vi "My Nonlinear Curve Fit TRDL bounds.vi"(0 "Y":dbl[](array[numeric]), 1 "f(x,a)":T4, 2 "data":variant, 5 "X":dbl[](array[numeric]), 7 "Weight":dbl[](array[numeric]), 9 "initial parameters":dbl[](array[numeric]), 11 "error in (no error)":errorcluster, 12 "termination":cluster{"max iteration":i32, "tolerance":dbl}={"max iteration"=200, "tolerance"=1e-08}, 13 "parameter bounds":T3, 14 "method":T2 items=["Least Square", "Least Absolute Residual", "Bisquare"]) -> (3 "Fit Aborted?":bool, 4 "best nonlinear fit":dbl[](array[numeric]), 6 "best fit parameters":dbl[](array[numeric]), 8 "covariance":T5, 10 "Fit Statistics":T1, 15 "error out":errorcluster)   [LabVIEW 2019]
uses:
  <vilib>/Analysis/Matrix/Datatypes/RealMatrix.ctl
  <vilib>/gmath/NumericalOptimization/LM model function reference.ctl
  <vilib>/Analysis/6fits.llb/Curve Fitting Criteria.ctl
  Fit Statistics.ctl
  <vilib>/gmath/NumericalOptimization/LM model function.ctl
  My Fit Stopping Criteria.ctl
  <vilib>/gmath/NumericalOptimization/LM_output select.ctl
  Abort Fit Global.vi
  <vilib>/gmath/NI_Gmath.lvlib
  <vilib>/Analysis/NI_AALBase.lvlib
  <vilib>/Analysis/Matrix/NI_Matrix.lvlib
  <vilib>/Analysis/NI_AALPro.lvlib
panel:
  out "Waveform Graph":dbl[](graph)
  in  "Delay (ms)":i32
  in  "Debug":bool
  out "Parameters Chart":dbl[][](graph)
  out "Function & Fit Graph":cluster{"New Coefficients":dbl[]}[](graph)
  in  "TR update constants":cluster{"h1":dbl, "h2":dbl, "a1":dbl, "a2":dbl}={"h1"=0.0001, "h2"=0.99, "a1"=0.25, "a2"=3.5}
  out "number of function calls":i32
  out "residue":dbl
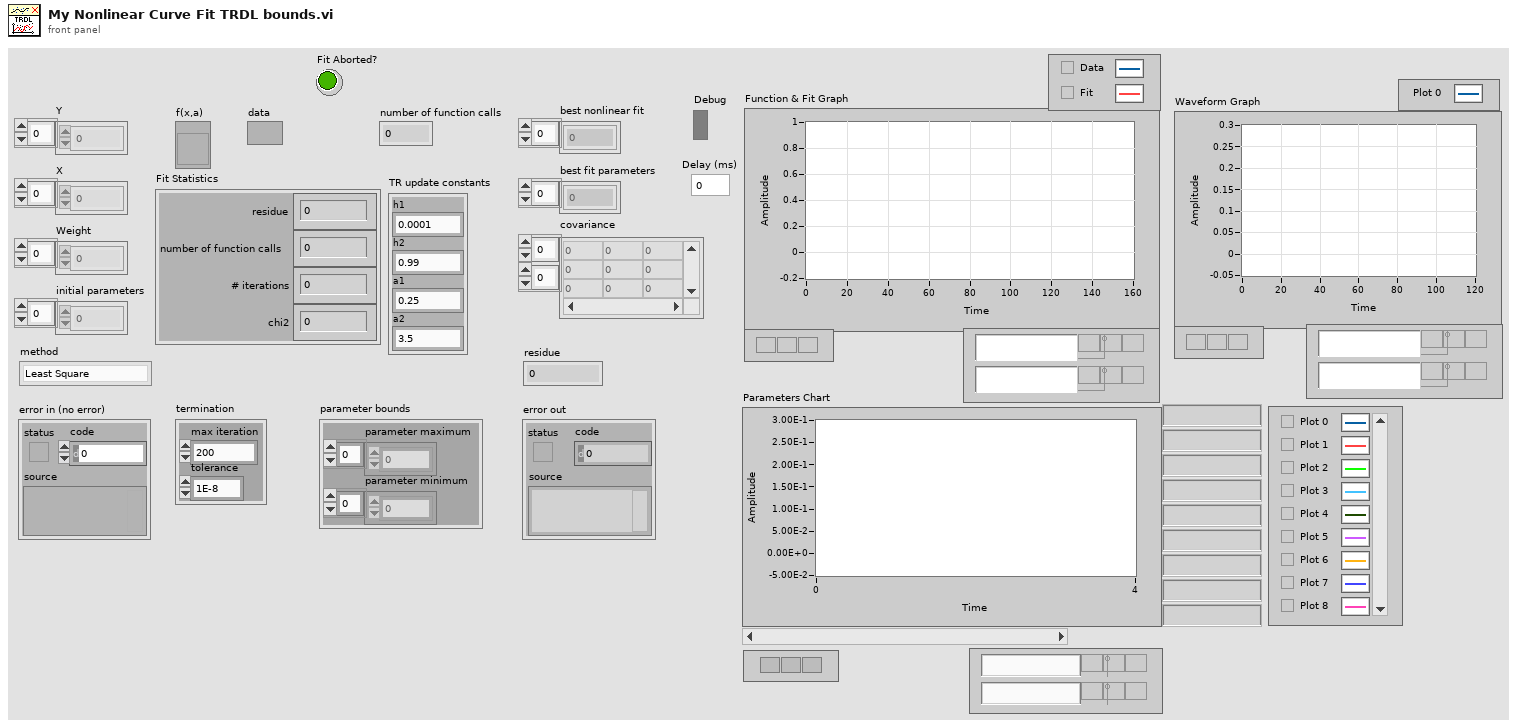
[diagram p1: front panel]
types:
  T1 = typedef "Fit Statistics.ctl" = cluster{"# iterations":i32, "number of function calls":i32, "chi2":dbl, "residue":dbl}
  T2 = typedef "NI_AALPro.lvlib/Curve Fitting Criteria.ctl" = u16
  T3 = cluster{"parameter minimum":dbl[], "parameter maximum":dbl[]}
  T4 = typedef "NI_Gmath.lvlib/LM model function reference.ctl" = refnum<vi>
  T5 = typedef "NI_Matrix.lvlib/RealMatrix.ctl" = dbl[][]
  T6 = typedef "My Fit Stopping Criteria.ctl" = cluster{"function tolerance":dbl, "parameter tolerance":dbl, "max iterations":i32, "max function calls":i32, "gradient tolerance":dbl, "max time (sec)":dbl, "initial tick count":u32, "min lambda":dbl, "max lambda":dbl}
  T7 = typedef "NI_Gmath.lvlib/LM model function.ctl" = cluster{"f(x,a)":T4, "data":variant}
  T8 = typedef "NI_Gmath.lvlib/LM_output select.ctl" = cluster{"model function":bool, "gradient":bool}
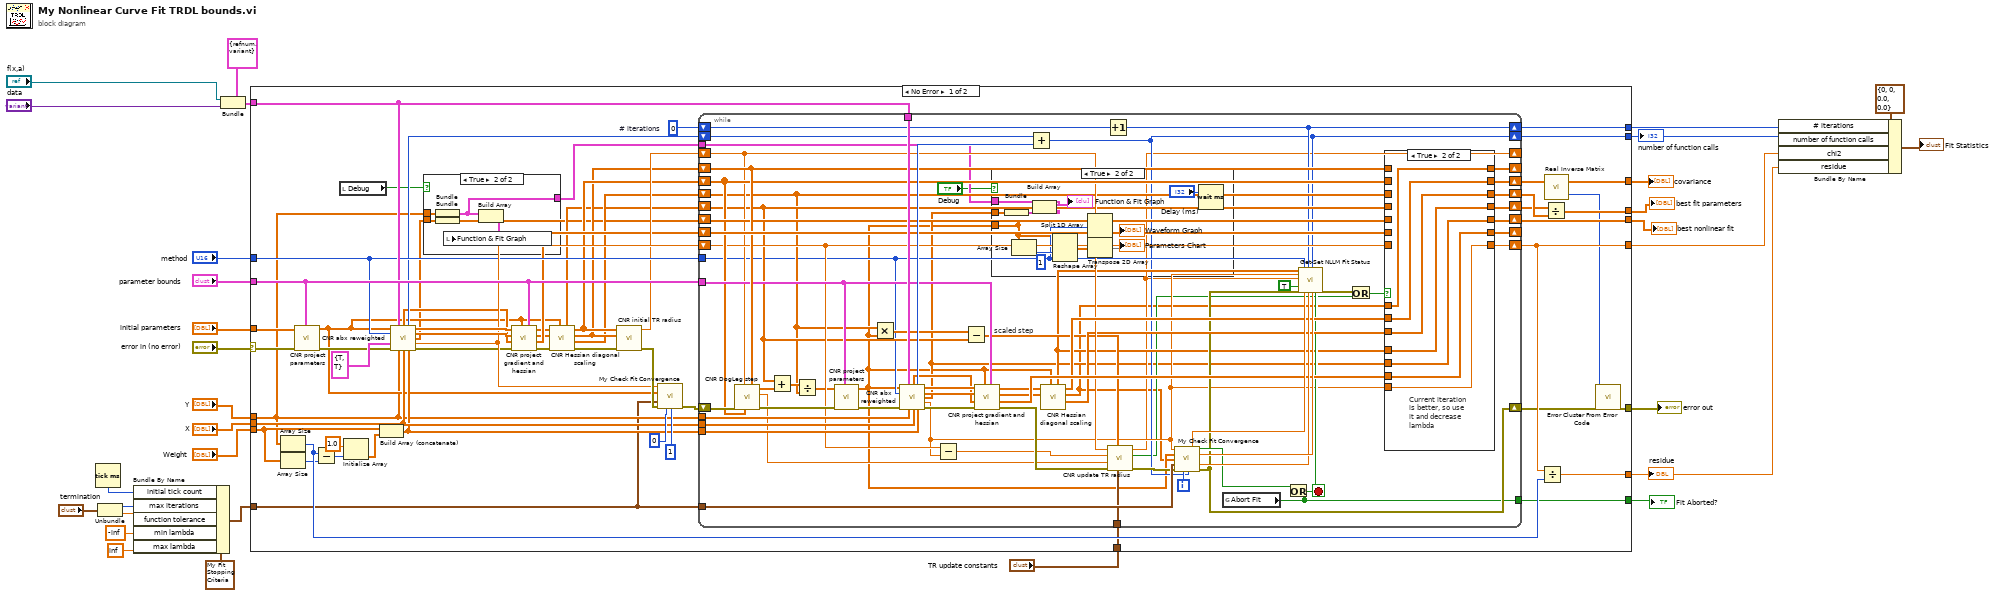
[diagram p0: block diagram]
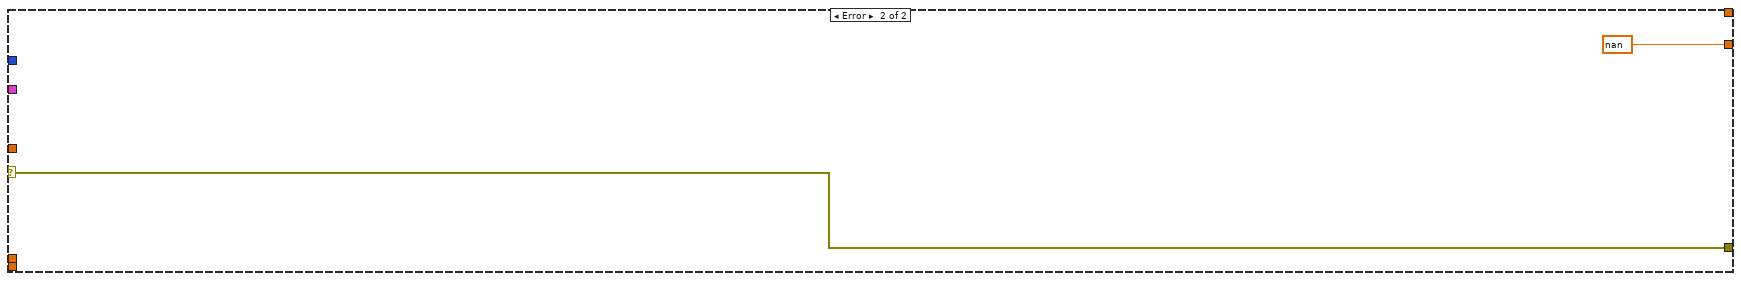
[diagram p5: hidden frame]
diagram:
  n1 = Tick Count (ms)() -> (millisecond timer value=w3:u32)
  n2 = Unbundle("termination") -> ("max iteration"=w21:i32, "tolerance"=w12:dbl)
  n3 = Bundle By Name(cluster=T6 {"function tolerance"=1e-06, "parameter tolerance"=100000000.0, "max iterations"=0, "max function calls"=1000000000, "gradient tolerance"=100000000.0, "max time (sec)"=-1.0, "initial tick count"=0, "min lambda"=1e-06, "max lambda"=1e-06} ("my stopping criteria"), "initial tick count"=w3, "max iterations"=w21, "function tolerance"=w12, "min lambda"=-inf, "max lambda"=inf) -> (w17:T6)
  n4 = Bundle(cluster=T7 {"f(x,a)"=refnum, "data"=variant} ("model function"), "f(x,a)"="f(x,a)", "data"="data") -> (w18:T7)
  n5 = case shown="No Error" "error in (no error)" {
    selector: "error in (no error)" -> [w72 w188]
    tunnel: [w44 _] -> w31
    tunnel: [w86 _] -> w7
    tunnel: "initial parameters" -> [w48 _]
    tunnel: [w58 _] -> w29
    tunnel: [w73 _] -> w28
    tunnel: "Weight" -> [w81 _]
    tunnel: "Y" -> [w34 _]
    tunnel: w17 -> [w32 _]
    tunnel: "X" -> [w60 _]
    tunnel: [w39 w188] -> w24
    tunnel: w18 -> [w66 _]
    tunnel: [w77 _] -> w8
    tunnel: "parameter bounds" -> [w71 _]
    tunnel: "method" -> [w65 _]
    tunnel: "TR update constants" -> [w57 _]
    tunnel: [w42 _] -> w10
    tunnel: [w41 nan ("chiSqr")] -> w6
    tunnel: [w37 _] -> w4
    frame No Error {
      w43 = 0  # # iterations
      n6 = Array Size(array=w34) -> (size(s)=w87:i32)
      n7 = Array Size(array=w81) -> (size(s)=w84:i32)
      n8 = call <vilib>:"CNR project parameters.vi"("bounds"=w71, "error in"=w72, "parameters"=w48) -> ("error out"=w64:errorcluster, "projected parameters"=w47:dbl[])  [unwired: 7 out]
      n9 = Subtract(x=w87, y=w84) -> (x-y=w83:i32)
      n10 = local read "Debug"() -> (w36:bool)
      n11 = Initialize Array(1.0, w83) -> (w82:dbl[])
      n12 = Build Array (concatenate)(w81, w82) -> (w59:dbl[])
      n13 = call <vilib>:"CNR abx reweighted.vi"("parameters"=w47, "model function"=w66, "method"=w65, "output control"=T8 {"model function"=TRUE, "gradient"=TRUE}, "error in (no error)"=w64, "Y"=w34, "X"=w60, "Weight"=w59) -> ("Jacobian"=w55:T5, "number of function calls"=w63:i32, "Hessian"=w70:T5, "gradient"=w69:dbl[], "best fit"=w35:dbl[], "chiSqr"=w68:dbl, "error out"=w62:errorcluster)  [unwired: 1 in]
      n14 = case shown="True" w36 {
        tunnel: w35 -> [_ w91]
        tunnel: w34 -> [_ w90]
        tunnel: [_ w88] -> w33
        frame False {
        }
        frame True {
          n15 = Bundle("Y"=w90) -> (w88:cluster{"Y":dbl[]})  [unwired: 1 in]
          n16 = Bundle("best fit"=w91) -> (w92:cluster{"best fit":dbl[]})  [unwired: 1 in]
          n17 = Build Array(w88, w92) -> (w89:cluster{"best fit":dbl[]}[])
          n18 = local write "Function & Fit Graph"(w89) -> ()
        }
      }
      n19 = call <vilib>:"CNR project gradient and hessian.vi"("bounds"=w71, "projected parameters"=w47, "error in"=w62, "Jacobian"=w55, "gradient"=w69, "Hessian"=w70) -> ("error out"=w61:errorcluster, "projected jacobian"=w54:T5, "projected gradient"=w51:dbl[], "projected Hessian"=w53:T5)  [unwired: 1 in, 1 out]
      n20 = call <vilib>:"CNR Hessian diagonal scaling.vi"("parameters"=w47, "gradient"=w51, "Hessian"=w53) -> ("D"=w49:dbl[], "scaled gradient"=w50:dbl[], "scaled Hessian"=w52:T5, "scaled parameters"=w46:dbl[])  [unwired: 5 out]
      n21 = call <vilib>:"CNR initial TR radius.vi"("error in"=w61, "g"=w50, "H"=w52) -> ("error out"=w75:errorcluster, "initial TR radius"=w56:dbl)  [unwired: 7 out]
      n22 = call "My Check Fit Convergence.vi"("Chi 2"=w68, "Parameters"=w47, "my stopping criteria"=w32, "Error In"=w75, "current iteration"=0, "number of function evaluations"=1) -> ("error out"=w80:errorcluster)  [unwired: 5 in, 4 out]
      n23 = while {
        tunnel: w60 -> [w157]
        tunnel: w34 -> [w133]
        shift-left: w68 -> [w128]
        shift-right: [w150] -> w41
        shift-left: w46 -> [w119]
        shift-right: [w147] -> w45
        shift-left: w56 -> [w120]
        shift-right: [w99] -> _
        shift-right: [w109] -> w40
        shift-left: w80 -> [w148]
        tunnel: w66 -> [w156]
        tunnel: w32 -> [w152]
        shift-right: [w103] -> w77
        shift-left: w63 -> [w155]
        shift-right: [w154] -> w58
        shift-left: w35 -> [w132]
        shift-right: [w151] -> _
        shift-left: w54 -> [w146]
        tunnel: w59 -> [w141]
        shift-right: [w145] -> w76
        shift-left: w49 -> [w113]
        tunnel: w71 -> [w134]
        shift-right: [w144] -> _
        shift-left: w50 -> [w142]
        shift-right: [w143] -> w74
        shift-left: w52 -> [w130]
        tunnel: w65 -> [w105]
        tunnel: w57 -> [w131]
        shift-right: [w104] -> w42
        shift-left: w43 -> [w111]
        tunnel: [w98] -> w37
        tunnel: w33 -> [w96]
        i -> [w153]
        stop <- w108 stop-if-true
        # "scaled step"
        n24 = call <vilib>:"CNR DogLeg step.vi"("gradient"=w142, "Hessian"=w130, "TR radius"=w120, "error in (no error)"=w148) -> ("error out"=w140:errorcluster, "L(0)-L(hdl)\npredicted change"=w123:dbl, "x step"=w117:dbl[])  [unwired: 3 in, 2 out]
        n25 = Add(x=w119, y=w117) -> (x+y=w116:dbl[])
        n26 = Divide(x=w116, y=w113) -> (x/y=w115:dbl[])
        n27 = call <vilib>:"CNR project parameters.vi"("bounds"=w134, "error in"=w140, "parameters"=w115) -> ("error out"=w139:errorcluster, "projected parameters"=w94:dbl[])  [unwired: 7 out]
        n28 = Multiply(x=w113, y=w94) -> (x*y=w112:dbl[])
        n29 = call <vilib>:"CNR abx reweighted.vi"("parameters"=w94, "model function"=w156, "method"=w105, "error in (no error)"=w139, "Y"=w133, "X"=w157, "Weight"=w141) -> ("Jacobian"=w122:T5, "number of function calls"=w158:i32, "Hessian"=w136:T5, "gradient"=w135:dbl[], "best fit"=w97:dbl[], "chiSqr"=w106:dbl, "error out"=w138:errorcluster)  [unwired: 2 in]
        n30 = Subtract(x=w128, y=w106) -> (x-y=w124:dbl)
        n31 = Subtract(x=w112, y=w119) -> (x-y=w114:dbl[])
        n32 = call <vilib>:"CNR project gradient and hessian.vi"("bounds"=w134, "projected parameters"=w94, "error in"=w138, "Jacobian"=w122, "gradient"=w135, "Hessian"=w136) -> ("error out"=w137:errorcluster, "projected jacobian"=w129:T5, "projected gradient"=w125:dbl[], "projected Hessian"=w127:T5)  [unwired: 1 in, 1 out]
        n33 = case shown="True" "Debug" {
          tunnel: w97 -> [_ w169]
          tunnel: w96 -> [_ w168]
          tunnel: w94 -> [_ w163]
          frame False {
          }
          frame True {
            w164 = 1 ("dimension size")
            n34 = Bundle("best fit"=w169) -> (w172:cluster{"best fit":dbl[]})  [unwired: 1 in]
            n35 = Array Size(array=w163) -> (size(s)=w171:i32)
            n36 = Build Array(w168, w172) -> (→"Function & Fit Graph":cluster{"best fit":dbl[]}[])
            n37 = Reshape Array(w163, w171, w164) -> (w170:dbl[][])
            n38 = Split 1D Array(array=w163, index=w164) -> (second subarray=→"Waveform Graph":dbl[])  [unwired: 1 out]
            n39 = Transpose 2D Array(2D array=w170) -> (transposed array=→"Parameters Chart":dbl[][])
            n40 = Wait (ms)(milliseconds to wait="Delay (ms)") -> ()  [unwired: 1 out]
          }
        }
        n41 = Add(x=w155, y=w158) -> (x+y=w103:i32)
        n42 = call <vilib>:"CNR Hessian diagonal scaling.vi"("parameters"=w94, "gradient"=w125, "Hessian"=w127) -> ("D"=w118:dbl[], "scaled gradient"=w93:dbl[], "scaled Hessian"=w126:T5, "scaled parameters"=w107:dbl[])  [unwired: 5 out]
        n43 = Increment(x=w111) -> (x+1=w104:i32)
        n44 = call <vilib>:"CNR update TR radius.vi"("TR update constants"=w131, "step"=w114, "error in (no error)"=w137, "L(0)-L(p_dl)"=w123, "F(x)-F(x+p)"=w124, "TR Radius"=w120) -> ("error out"=w149:errorcluster, "step OK?"=w101:bool, "TR Radius out"=w99:dbl)  [unwired: 3 out]
        n45 = call "My Check Fit Convergence.vi"("Chi 2"=w106, "Parameters"=w94, "gradient"=w93, "my stopping criteria"=w152, "Error In"=w149, "current iteration"=w153, "number of function evaluations"=w103) -> ("|Delta Chi 2|/Chi 2"=w161:dbl, "stop?"=w121:bool, "|Delta Chi 2|"=w160:dbl, "Max |Delta a| /|a|"=w159:dbl, "error out"=w109:errorcluster)  [unwired: 4 in]
        n46 = global read "Abort Fit Global.vi" "Abort Fit"() -> (w98:bool)
        n47 = Or(x=w121, y=w98) -> (x .or. y?=w108:bool)
        n48 = call "Get-Set NLLM Fit Status.vi"("Fit Parameters"=w107, "chiSqr"=w106, "Lambda"=w99, "Get(F)/Set"=TRUE, "Error In"=w109, "method"=w105, "|Delta Chi 2|/Chi 2"=w161, "# Iterations"=w104, "Max |Delta a| /|a|"=w159, "# Function Calls"=w103, "|Delta Chi 2|"=w160, "Done"=w108) -> ("Error Out"=w102:errorcluster)  [unwired: 6 in, 1 out]
        n49 = Or(x=w102, y=w101) -> (x .or. y?=w100:bool)
        n50 = case shown="True" w100 {
          tunnel: w107 -> [_ w180]
          tunnel: w119 -> [w179 _]
          tunnel: [w179 w180] -> w147
          tunnel: w128 -> [w178 _]
          tunnel: w106 -> [_ w186]
          tunnel: [w178 w186] -> w150
          tunnel: w132 -> [w177 _]
          tunnel: [w177 w184] -> w154
          tunnel: w146 -> [w176 _]
          tunnel: [w176 w185] -> w151
          tunnel: w129 -> [_ w185]
          tunnel: w97 -> [_ w184]
          tunnel: w113 -> [w175 _]
          tunnel: [w175 w181] -> w145
          tunnel: w142 -> [w174 _]
          tunnel: w130 -> [w173 _]
          tunnel: [w174 w183] -> w144
          tunnel: [w173 w182] -> w143
          tunnel: w93 -> [_ w183]
          tunnel: w126 -> [_ w182]
          tunnel: w118 -> [_ w181]
          frame False {
            # "Previous iteration\nis better, so keep\nit and increase \nlambda"
          }
          frame True {
            # "Current iteration\nis better, so use\nit and decrease \nlambda"
          }
        }
      }
      n51 = Divide(x=w41, y=w87) -> (x/y=w86:dbl)
      n52 = Divide(x=w45, y=w76) -> (x/y=w44:dbl[])
      n53 = call <vilib>:"Real Inverse Matrix.vi"("Input Matrix"=w74) -> ("error"=w38:i32, "Inverse Matrix"=w73:T5)  [unwired: 1 in]
      n54 = call <vilib>:"Error Cluster From Error Code.vi"("error in (no error)"=w40, "error code (0)"=w38) -> ("error out"=w39:errorcluster)  [unwired: 1 in, 6 out]
    }
    frame Error {
    }
  }
  "residue" <- w7
  "best fit parameters" <- w31
  "best nonlinear fit" <- w29
  "error out" <- w24
  "covariance" <- w28
  "number of function calls" <- w8
  "Fit Aborted?" <- w4
  n55 = Bundle By Name(cluster=T1 {"# iterations"=0, "number of function calls"=0, "chi2"=0.0, "residue"=0.0} ("Fit Statistics"), "# iterations"=w10, "number of function calls"=w8, "chi2"=w6, "residue"=w7) -> (→"Fit Statistics":T1)
